vi "COMI DIO Set Usage.vi"(10 "usage":i32, 11 "hDevice":u32) -> (3 "hDevice out":u32)   [LabVIEW 2017, in "Comidll.lvlib"]
doc: "void (COMI_DIO_SetUsage) (HANDLE hDevice, int usage);"
uses:
  <userlib>/Comidll/Comidll.lvlib
  <userlib>/Comidll/Comidll.dll
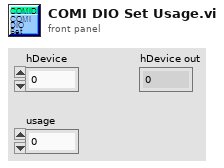
[diagram p1: front panel]
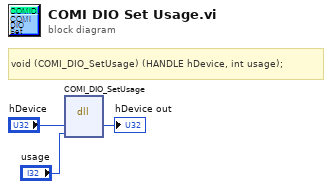
[diagram p0: block diagram]
diagram:
  # "void\t(COMI_DIO_SetUsage) (HANDLE hDevice, int usage);"
  n1 = dll-call lib="C:/Program Files/National Instruments/LabVIEW 2017/user.lib/Comidll/Comidll.*" fn="COMI_DIO_SetUsage"("hDevice"="hDevice", "usage"="usage") -> ("hDevice"=→"hDevice out":u32)  [unwired: 5 in, 2 out]
